vi "Info from Source.vi"(8 "error in (no error)":errorcluster, 9 "Branch (Default)":string, 10 "Source":string, 11 "GitPackage in":refnum<class "GitPackage.lvclass">) -> (0 "error out":errorcluster, 2 "Package Info":T1, 3 "GitPackage out":refnum<class "GitPackage.lvclass">)   [LabVIEW 2020, in "GPack.lvlib" / "GitPackage.lvclass"]
uses:
  GitPackage.lvclass
  Package Info.ctl
  <vilib>/Hampel Software Engineering/Git API/Git API/GIT-api.lvclass
  GPack.lvlib
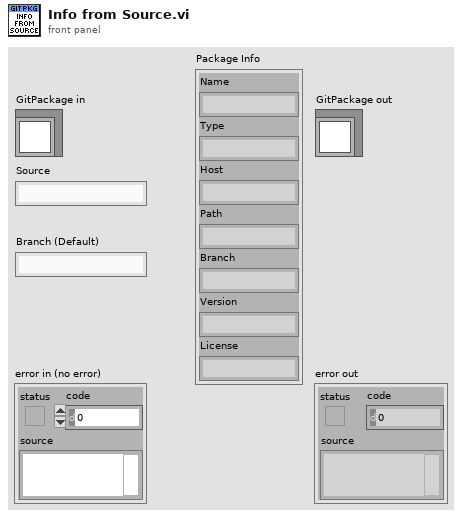
[diagram p1: front panel]
types:
  T1 = typedef "GPack.lvlib/Package Info.ctl" = cluster{"Name":string, "Type":string, "Host":string, "Path":string, "Branch":string, "Version":string, "License":string}
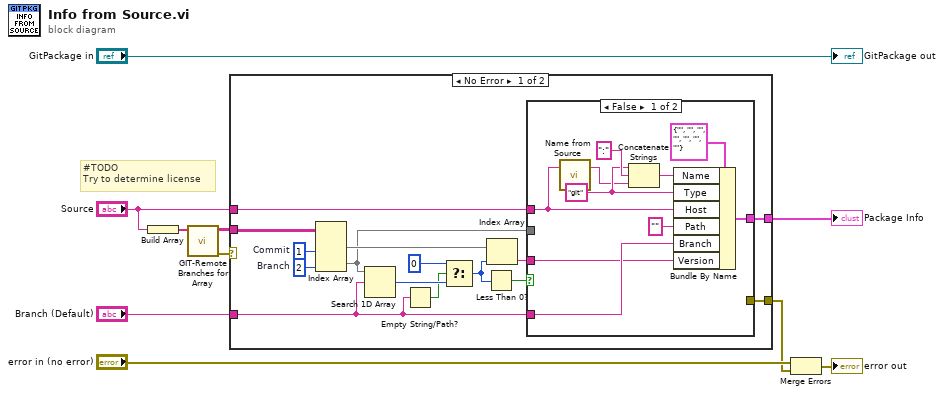
[diagram p0: block diagram]
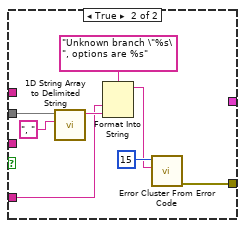
[diagram p2: hidden frame]
diagram:
  # "#TODO\nTry to determine license"
  n1 = Build Array("Source") -> (w8:string[])
  n2 = call <vilib>:"GIT-Remote Branches for Array.vi"("remotes"=w8) -> ("error out"=w7:errorcluster, "branches"=w6:string[][])  [unwired: 9 in]
  n3 = case shown="No Error" w7 {
    selector: w7 -> [_ w44]
    tunnel: w6 -> [w25 _]
    tunnel: "Branch (Default)" -> [w16 _]
    tunnel: "Source" -> [w19 _]
    tunnel: [w18 _] -> w3
    tunnel: [w11 w44] -> w1
    frame No Error {
      w23 = 1  # Commit
      w24 = 2  # Branch
      n4 = Index Array(array=w25, index (col) #1=w23, index (col) #2=w24) -> (element #1=w22:string[], element #2=w17:string[])  [unwired: 2 in]
      n5 = Search 1D Array(1D array=w17, element=w16) -> (index of element=w15:i32)  [unwired: 1 in]
      n6 = Empty String/Path?(string/path=w16) -> (empty?=w12:bool)
      n7 = Select(t=0, s=w12, f=w15) -> (s? t:f=w13:i32)
      n8 = Less Than 0?(x=w13) -> (x < 0?=w21:bool)
      n9 = Index Array(array=w22, index=w13) -> (element=w20:string)
      n10 = case shown="False" w21 {
        tunnel: w20 -> [w31 _]
        tunnel: w16 -> [w32 w38]
        tunnel: w19 -> [w34 _]
        tunnel: [w30 _] -> w18
        tunnel: w17 -> [_ w41]
        tunnel: [_ w36] -> w11
        frame False {
          w27 = "git" ("Type")
          n11 = call "Name from Source.vi"("Source"=w34) -> ("Name"=w26:string)  [unwired: 2 in]
          n12 = Concatenate Strings(w27, ":" ("string"), w26) -> (w29:string)
          n13 = Bundle By Name(cluster=T1 {"Name"="", "Type"="", "Host"="", "Path"="", "Branch"="", "Version"="", "License"=""} ("Package Info"), "Name"=w29, "Type"=w27, "Host"=w34, "Path"="", "Branch"=w32, "Version"=w31) -> (w30:T1)
        }
        frame True {
          n14 = call <vilib>:"1D String Array to Delimited String.vi"("delimiter"=", ", "string array"=w41) -> ("delimited string"=w39:string)  [unwired: 9 in]
          n15 = Format Into String(format string="Unknown branch \"%s\", options are %s", w38, w39) -> (resulting string=w37:string)  [unwired: 2 in, 1 out]
          n16 = call <vilib>:"Error Cluster From Error Code.vi"("error message (\"\")"=w37, "error code (0)"=15) -> ("error out"=w36:errorcluster)  [unwired: 7 in]
        }
      }
    }
    frame Error {
    }
  }
  "Package Info" <- w3
  n17 = Merge Errors("error in (no error)", w1) -> (→"error out":errorcluster)
  "GitPackage out" <- "GitPackage in"
